vi "P4CMD Run Provider.vi"(8 "error in (no error)":errorcluster) -> (0 "error out":errorcluster)   [LabVIEW 2017, in "NI_SCC_P4CMD.lvlib"]
uses:
  <vilib>/SourceControl/Providers/P4CMD/NI_SCC_P4CMD.lvlib
  <vilib>/SourceControl/support/SCCSup Message Strings GLBL.vi
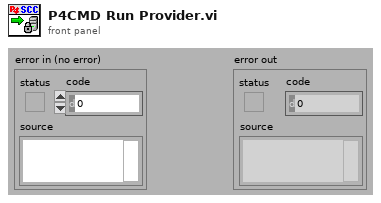
[diagram p1: front panel]
types:
  T1 = enum32{"invalid OS target", "Mac OS", "Windows 3.1", "Windows 95/NT", "Solaris 1", "Solaris 2", "HP-UX", "PowerMAX", "Linux", "Irix", "Rhapsody", "BeOS", "AIX", "OSF1", "VxWorks", "PharLap", "Carbon", "RTX", "Windows x64", "Linux x64", "Mac OS X x64"}
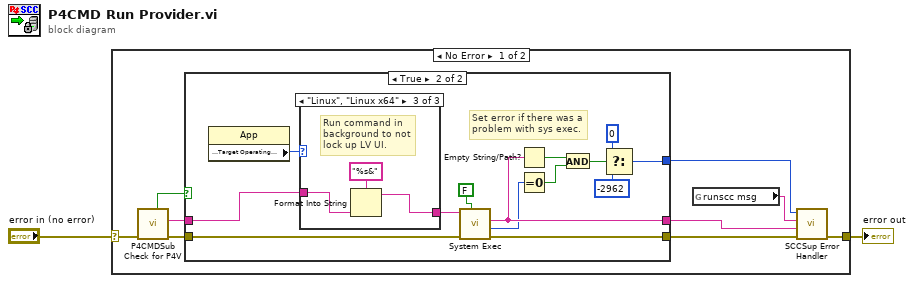
[diagram p0: block diagram]
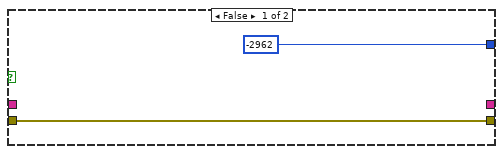
[diagram p2: hidden frame]
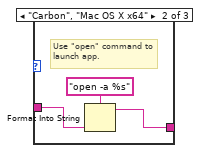
[diagram p4: hidden frame]
diagram:
  n1 = case shown="No Error" "error in (no error)" {
    selector: "error in (no error)" -> [w8 w35]
    tunnel: [w11 w35] -> w1
    frame No Error {
      n2 = call <vilib>:"P4CMDSub Check for P4V.vi"("error in (no error)"=w8) -> ("error out"=w6:errorcluster, "visual client path"=w5:string, "visual client found?"=w4:bool)  [unwired: 8 in]
      n3 = case shown="True" w4 {
        tunnel: [w13 w27] -> w9
        tunnel: [_ w19] -> w7
        tunnel: w6 -> [w13 w25]
        tunnel: w5 -> [_ w24]
        tunnel: [-2962 ("error code") w15] -> w3
        frame False {
        }
        frame True {
          # "Set error if there was a problem with sys exec."
          n4 = property class="App"() -> ("Application:Target Operating System"=w23:T1)  [unwired: 2 in, 2 out]
          n5 = case shown="\"Linux\", \"Linux x64\"" w23 {
            tunnel: w24 -> [w28 w30 w33]
            tunnel: [w28 w29 w32] -> w22
            frame Default {
            }
            frame "Carbon", "Mac OS X x64" {
              # "Use \"open\" command to launch app."
              n6 = Format Into String(format string="open -a %s" ("visual client path"), w30) -> (resulting string=w29:string)  [unwired: 2 in, 1 out]
            }
            frame "Linux", "Linux x64" {
              # "Run command in background to not lock up LV UI."
              n7 = Format Into String(format string="%s&" ("visual client path"), w33) -> (resulting string=w32:string)  [unwired: 2 in, 1 out]
            }
          }
          n8 = call <vilib>:"System Exec.vi"("wait until completion? (T)"=FALSE, "error in (no error)"=w25, "command line"=w22) -> ("error out"=w27:errorcluster, "return code"=w18:i32, "standard error"=w19:string)  [unwired: 5 in, 1 out]
          n9 = Empty String/Path?(string/path=w19) -> (empty?=w21:bool)
          n10 = Equal To 0?(x=w18) -> (x = 0?=w20:bool)
          n11 = And(x=w21, y=w20) -> (x .and. y?=w17:bool)
          n12 = Select(t=0 ("error code"), s=w17, f=-2962 ("error code")) -> (s? t:f=w15:i32)
        }
      }
      n13 = global read "SCCSup Message Strings GLBL.vi" "runscc msg"() -> (w10:string)
      n14 = call <vilib>:"SCCSup Error Handler.vi"("error in (no error)"=w9, "additional message"=w7, "operation message"=w10, "scc error code"=w3) -> ("error out"=w11:errorcluster)  [unwired: 7 in]
    }
    frame Error {
    }
  }
  "error out" <- w1
